vi "cmc_Epitrochoid.vi"() -> ()   [LabVIEW 2010]
uses:
  <vilib>/express/express arith-compare/Formula/XNode/ExpressFormulaBlockNode.xnode
panel:
  out "XY Graph":cluster{dbl[], dbl[]}(graph)
  out "Waveform Graph":cluster{dbl, dbl, dbl[][]}(graph)
  in  "Delay Time (s)":dbl=0.001
  out "Waveform Chart":cluster{"Result":dbl, "Result":dbl}(graph)={"Result"=0.4836981066564806, "Result"=35.62422485295828}
  in  "Generatrix h:":dbl=13.0
  in  "Major Radius a:":dbl=18.0
  in  "Minor Radius b:":dbl=8.0
  in  "Periods:":u8=10
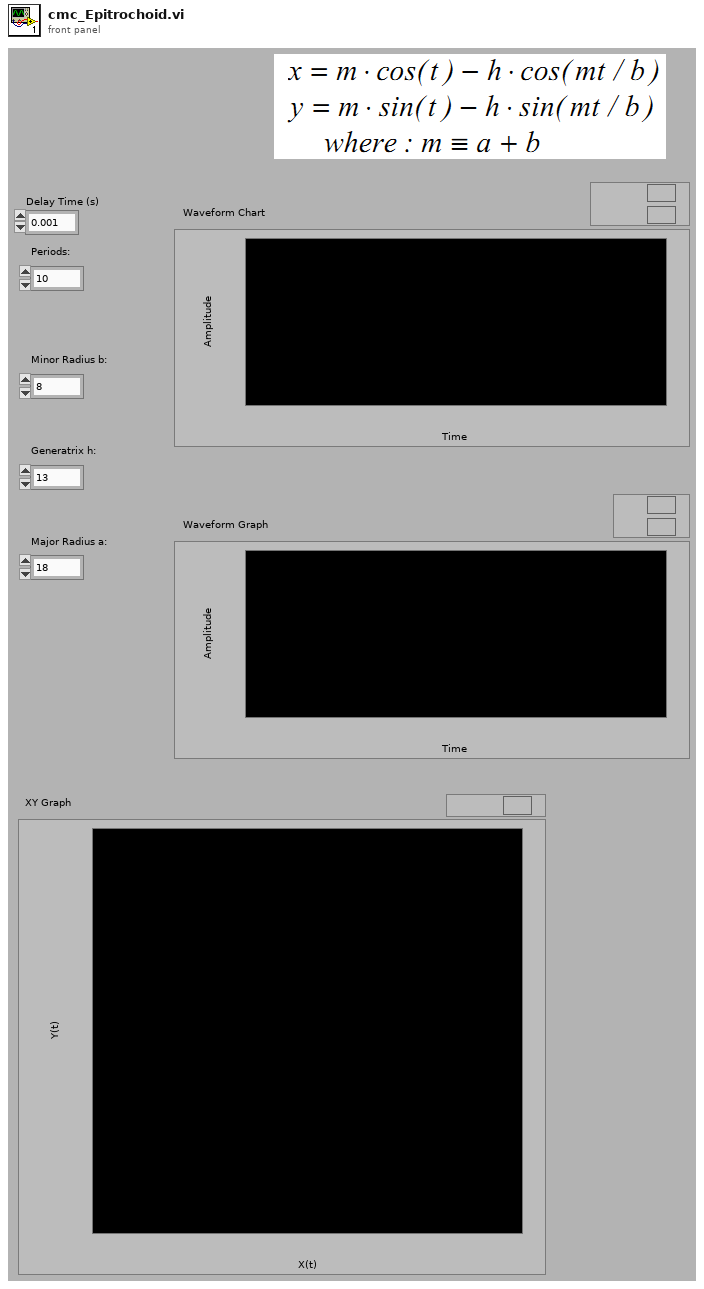
[diagram p1: front panel]
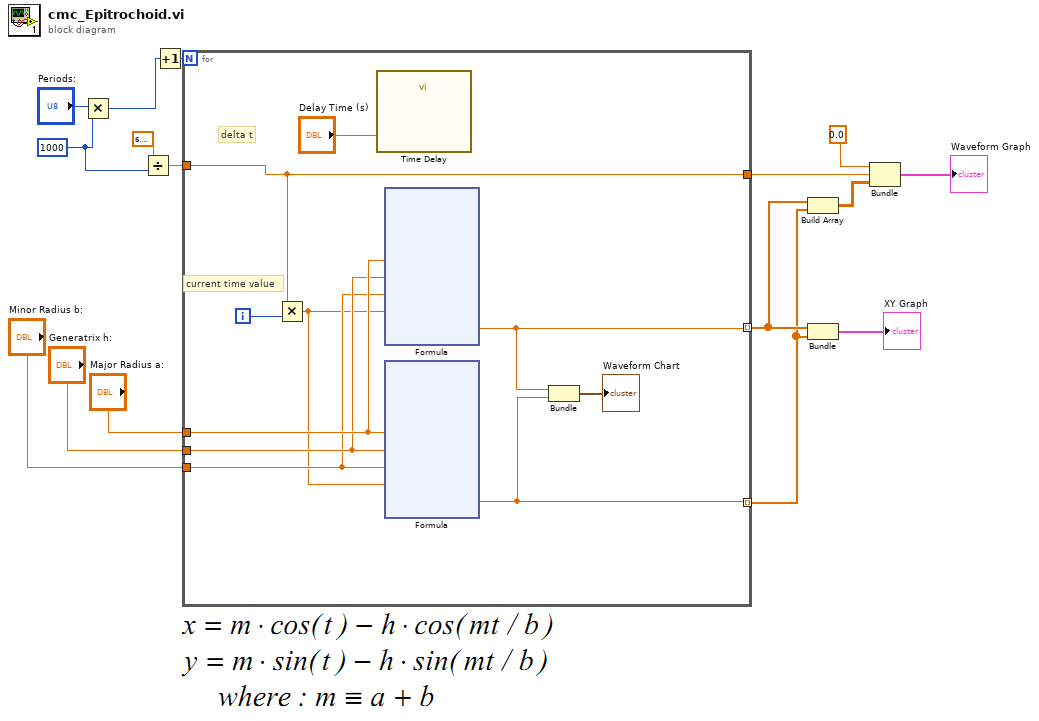
[diagram p0: block diagram]
diagram:
  w8 = 1000
  n1 = Multiply(x="Periods:", y=w8) -> (x*y=w13:i32)
  n2 = Divide(x=6.283185307179586, y=w8) -> (x/y=w12:dbl)
  n3 = Increment(x=w13) -> (x+1=w15:i32)
  n4 = for {
    N: w15 -> [_]
    tunnel: w12 -> [w21]
    tunnel: "Major Radius a:" -> [w25]
    tunnel: "Generatrix h:" -> [w24]
    tunnel: "Minor Radius b:" -> [w23]
    tunnel: [w21] -> w7
    tunnel: [w18] -> w3 mode=indexing
    tunnel: [w17] -> w2 mode=indexing
    i -> [w26]
    # "current time value"
    # "delta t"
    n5 = Multiply(x=w21, y=w26) -> (x*y=w22:dbl)
    n6 = call "Time Delay"("Delay Time (s)"="Delay Time (s)") -> ()  [unwired: 10 in, 1 out]
    n7 = xnode "Formula"("a"=w25, "h"=w24, "b"=w23, "t"=w22) -> ("Result"=w18:dbl)  [unwired: 1 in, 1 out]
    n8 = xnode "Formula"("a"=w25, "h"=w24, "b"=w23, "t"=w22) -> ("Result"=w17:dbl)  [unwired: 1 in, 1 out]
    n9 = Bundle("Result"=w18, "Result"=w17) -> (→"Waveform Chart":cluster{"Result":dbl, "Result":dbl})  [unwired: 1 in]
  }
  n10 = Build Array(w3, w2) -> (w5:dbl[][])
  n11 = Bundle(w3, w2) -> (→"XY Graph":cluster{dbl[], dbl[]})  [unwired: 1 in]
  n12 = Bundle(0.0, w7, w5) -> (→"Waveform Graph":cluster{dbl, dbl, dbl[][]})  [unwired: 1 in]
